vi "zad8.vi"(7 "Wartosc max":dbl, 8 "error in (no error)":errorcluster, 9 "Wartosc min":dbl, 10 "x":dbl[](array[numeric]), 11 "n":u32) -> (0 "error out":errorcluster)   [LabVIEW 2017]
panel:
  out "Wartoœæ":dbl
  out "wspolczynniki wielomianu":dbl[](array[numeric])
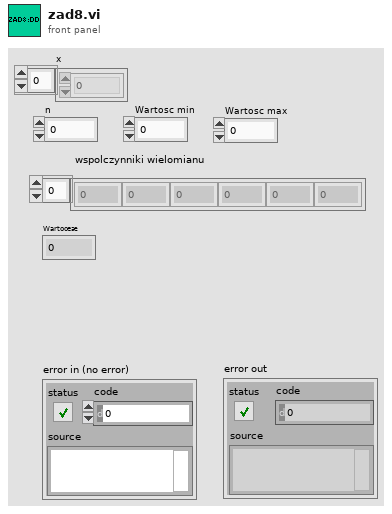
[diagram p1: front panel]
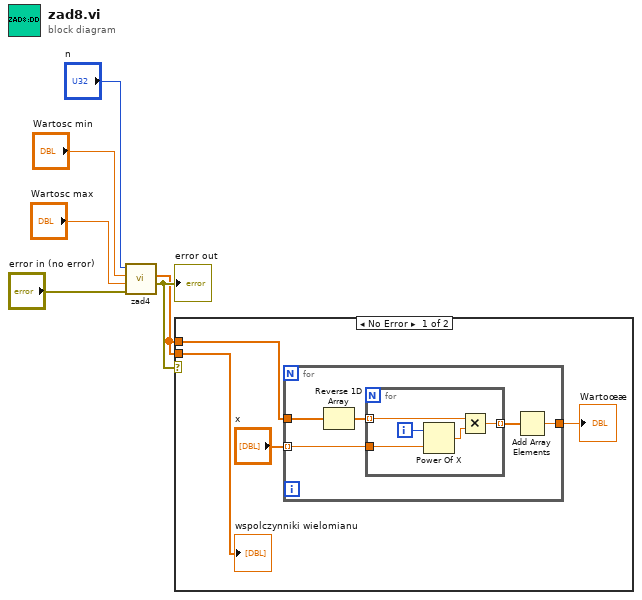
[diagram p0: block diagram]
diagram:
  n1 = call "zad4.vi"("error in (no error)"="error in (no error)", "Max"="Wartosc max", "Min"="Wartosc min", "N"="n") -> ("error out"=w2:errorcluster, "Array"=w1:dbl[])  [unwired: 6 in]
  "error out" <- w2
  n2 = case shown="No Error" w2 {
    tunnel: w1 -> [w9 _]
    tunnel: w1 -> [w8 _]
    frame No Error {
      n3 = for {
        tunnel: "x" -> [w15] mode=indexing
        tunnel: w9 -> [w13]
        tunnel: [w11] -> w7
        n4 = Reverse 1D Array(array=w13) -> (reversed array=w14:dbl[])
        n5 = for {
          tunnel: w14 -> [w16] mode=indexing
          tunnel: w15 -> [w19]
          tunnel: [w17] -> w12 mode=indexing
          i -> [w20]
          n6 = Power Of X(1:w19, 2:w20) -> (0:w18:dbl)
          n7 = Multiply(x=w16, y=w18) -> (x*y=w17:dbl)
        }
        n8 = Add Array Elements(numeric array=w12) -> (sum=w11:dbl)
      }
      "Wartoœæ" <- w7
      "wspolczynniki wielomianu" <- w8
    }
    frame Error {
    }
  }
